vi "log_main.vi"(7 "FGV_mods":T1, 8 "Error In":errorcluster, 11 "DataIn":variant) -> (0 "Error Out":errorcluster, 3 "DataOut":variant)   [LabVIEW 2016]
uses:
  log_mods.ctl
  log_data.ctl
  log_status.ctl
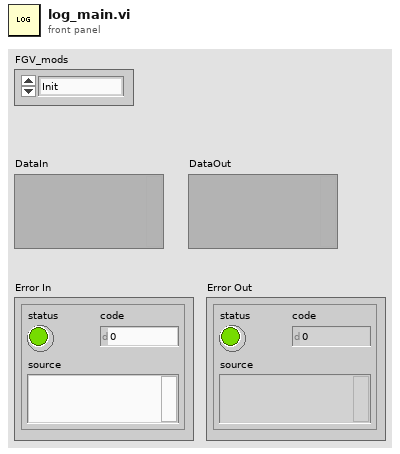
[diagram p1: front panel]
types:
  T1 = typedef "log_mods.ctl" = enum16{"Init", "LogFileRefnum", "SetStatus", "WriteSG", "WriteCM", "WriteToLog", "End"}
  T2 = typedef "log_data.ctl" = cluster{"log_status":T3, "SG_data":dbl[], "CM_data":dbl[], "LogRef":refnum<vi>, "log_file":refnum<file>}
  T3 = typedef "log_status.ctl" = enum16{"Init", "Ready", "Running", "Error", "End"}
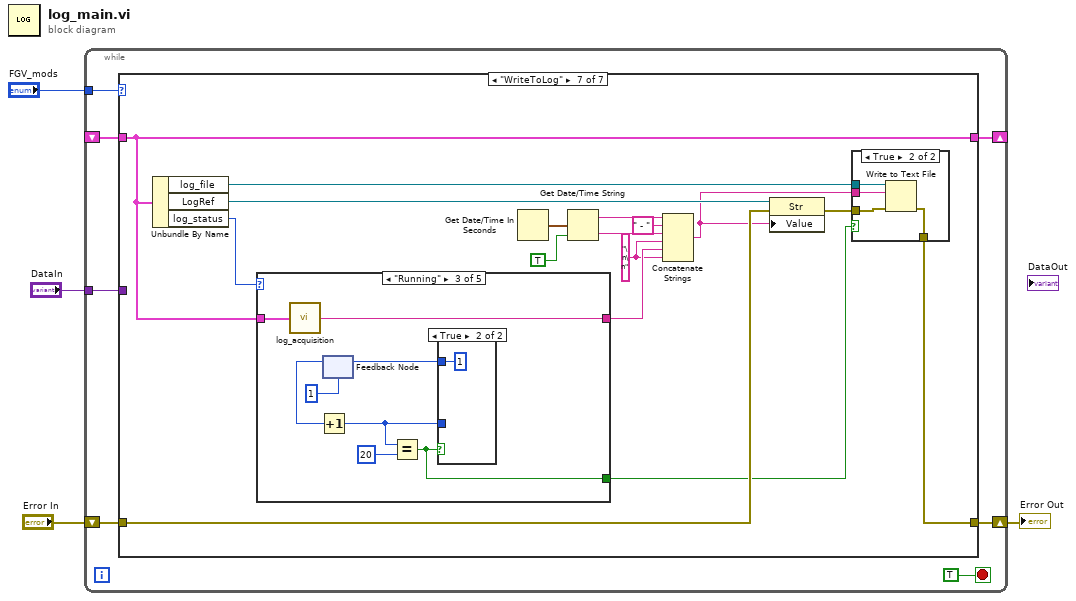
[diagram p0: block diagram]
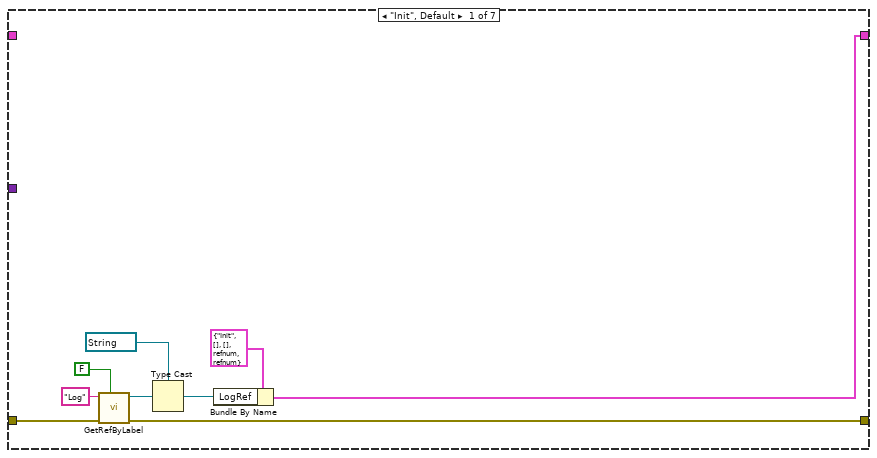
[diagram p2: hidden frame]
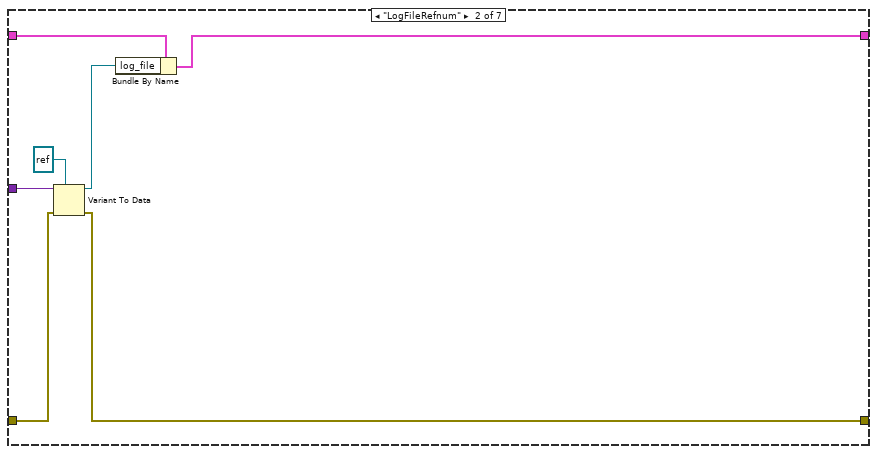
[diagram p3: hidden frame]
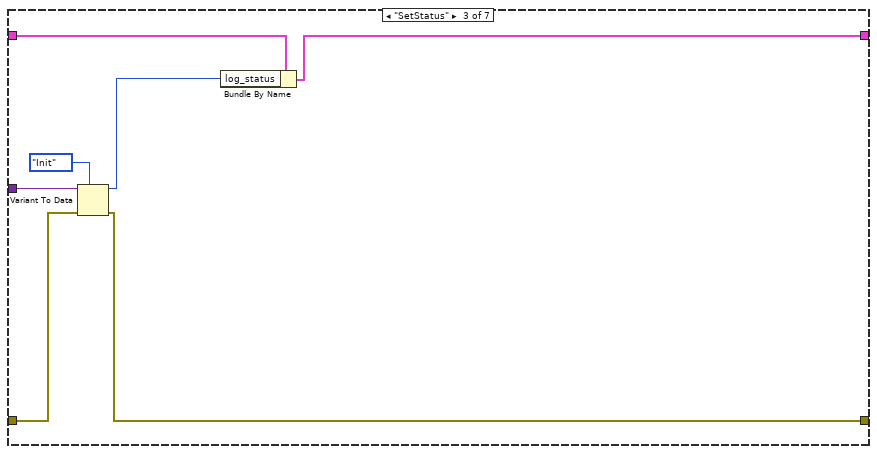
[diagram p4: hidden frame]
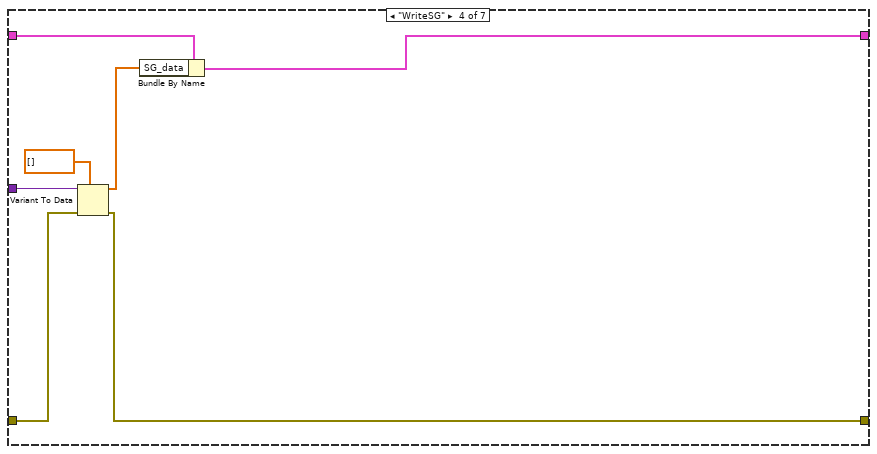
[diagram p5: hidden frame]
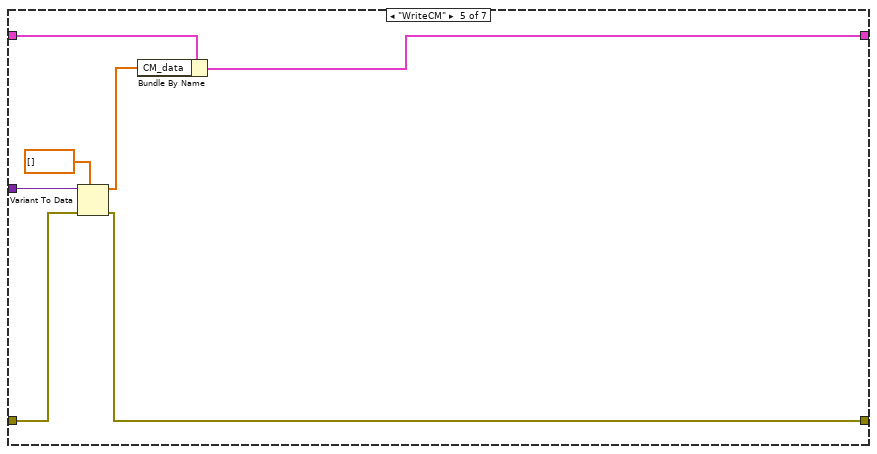
[diagram p6: hidden frame]
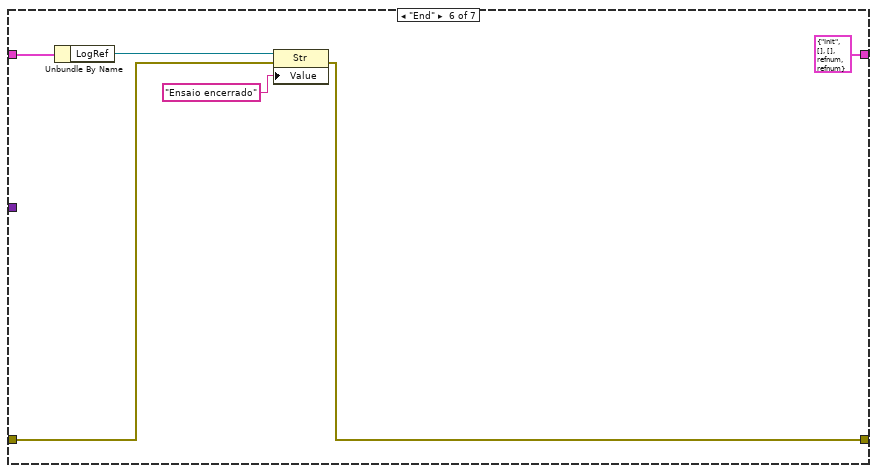
[diagram p7: hidden frame]
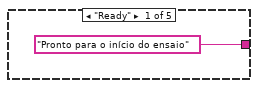
[diagram p9: hidden frame]
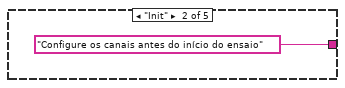
[diagram p10: hidden frame]
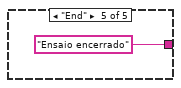
[diagram p13: hidden frame]
diagram:
  n1 = while {
    tunnel: "DataIn" -> [w10]
    tunnel: "FGV_mods" -> [w9]
    shift-right: [w8] -> _
    shift-left: _ -> [w7]
    shift-right: [w5] -> w1
    shift-left: "Error In" -> [w6]
    stop <- TRUE stop-if-true
    n2 = case shown="\"WriteToLog\"" w9 {
      tunnel: w10 -> [_ w26 w32 w39 w46 _ _]
      tunnel: [w13 w21 w33 w40 w47 T2 {"log_status"=enum."Init", "SG_data"=[], "CM_data"=[], "LogRef"=refnum, "log_file"=refnum} ("log_data") w69] -> w8
      tunnel: w7 -> [_ w23 w34 w41 w48 w53 w69]
      tunnel: w6 -> [w18 w25 w31 w38 w45 w50 w67]
      tunnel: [w12 w24 w28 w37 w44 w49 w56] -> w5
      frame "Init", Default {
        n3 = call "GetRefByLabel.vi"("InsideTab"=FALSE, "error in"=w18, "Label"="Log") -> ("error out"=w12:errorcluster, "Ctl Refnum"=w17:refnum<vi>)  [unwired: 6 in, 1 out]
        n4 = Type Cast(type=refnum<vi> refnum ("Log"), x=w17) -> (*(type *) &x=w14:refnum<vi>)
        n5 = Bundle By Name(cluster=T2 {"log_status"=enum."Init", "SG_data"=[], "CM_data"=[], "LogRef"=refnum, "log_file"=refnum} ("log_data"), "LogRef"=w14) -> (w13:T2)
      }
      frame "LogFileRefnum" {
        n6 = Variant To Data(error in=w25, type=refnum<file> refnum ("log_file"), Variant=w26) -> (data=w22:refnum<file>, error out=w24:errorcluster)
        n7 = Bundle By Name(cluster=w23, "log_file"=w22) -> (w21:T2)
      }
      frame "SetStatus" {
        n8 = Variant To Data(error in=w31, type=log_status."Init" ("log_status"), Variant=w32) -> (data=w29:T3, error out=w28:errorcluster)
        n9 = Bundle By Name(cluster=w34, "log_status"=w29) -> (w33:T2)
      }
      frame "WriteSG" {
        n10 = Variant To Data(error in=w38, type=dbl[] [] ("SG_data"), Variant=w39) -> (data=w35:dbl[], error out=w37:errorcluster)
        n11 = Bundle By Name(cluster=w41, "SG_data"=w35) -> (w40:T2)
      }
      frame "WriteCM" {
        n12 = Variant To Data(error in=w45, type=dbl[] [] ("SG_data"), Variant=w46) -> (data=w42:dbl[], error out=w44:errorcluster)
        n13 = Bundle By Name(cluster=w48, "CM_data"=w42) -> (w47:T2)
      }
      frame "End" {
        n14 = Unbundle By Name(w53) -> ("LogRef"=w52:refnum<vi>)
        n15 = property class="Str"(reference=w52, error in=w50, "Value"="Ensaio encerrado") -> (error out=w49:errorcluster)  [unwired: 1 out]
      }
      frame "WriteToLog" {
        w55 = "\n\n" ("string")
        n16 = Unbundle By Name(w69) -> ("log_file"=w58:refnum<file>, "LogRef"=w68:refnum<vi>, "log_status"=w70:T3)
        n17 = case shown="\"Running\"" w70 {
          tunnel: w69 -> [_ _ w85 _ _]
          tunnel: ["Pronto para o início do ensaio" ("Value") "Configure os canais antes do início do ensaio" ("Value") w84 _ "Ensaio encerrado" ("Value")] -> w62
          tunnel: [_ _ w78 _ _] -> w60
          frame "Ready" {
          }
          frame "Init" {
          }
          frame "Running" {
            n18 = call "log_acquisition.vi"("log_data"=w85) -> ("Log"=w84:string)
            n19 = feedback #1(1) -> (w83:i32)
            n20 = Increment(x=w83) -> (x+1=w79:i32)
            n21 = Equal?(x=w79, y=20) -> (x = y?=w78:bool)
            n22 = case shown="True" w78 {
              tunnel: [w86 1 ("y")] -> w80
              tunnel: w79 -> [w86 _]
              frame False {
              }
              frame True {
              }
            }
            n23 = feedback-in #1(w80) -> ()
          }
          frame "Error" {
          }
          frame "End" {
          }
        }
        n24 = Get Date/Time In Seconds() -> (seconds since 1Jan1904=w66:timestamp)
        n25 = Get Date/Time String(seconds (now)=w66, want seconds? (F)=TRUE) -> (date string=w65:string, time string=w64:string)  [unwired: 1 in]
        n26 = Concatenate Strings(w65, " - " ("string"), w64, w55, w62, w55) -> (w57:string)
        n27 = property class="Str"(reference=w68, error in=w67, "Value"=w57) -> (error out=w59:errorcluster)  [unwired: 1 out]
        n28 = case shown="True" w60 {
          tunnel: w59 -> [w71 w75]
          tunnel: w58 -> [_ w74]
          tunnel: w57 -> [_ w73]
          tunnel: [w71 w72] -> w56
          frame False {
          }
          frame True {
            n29 = Write to Text File(file (use dialog)=w74, text=w73, error in=w75) -> (error out=w72:errorcluster)  [unwired: 1 in, 2 out]
          }
        }
      }
    }
  }
  "Error Out" <- w1
